vi "Ramp Motors.vi"() -> ()   [LabVIEW 2018]
uses:
  <vilib>/Rock Robotics/WPI/ThirdParty/Phoenix-LabVIEW/Motor Controller/Controls/CTRE_Phoenix_MotorControl_NeutralMode.ctl
  <vilib>/Rock Robotics/WPI/ThirdParty/Phoenix-LabVIEW/Motor Controller/Controls/CTRE_Phoenix_MotorControl_ControlMode.ctl
  Framework/Robot Global Data.vi
  <vilib>/ptbypt/NI_PtbyPt.lvlib
panel:
  in  "Target Time (s)":dbl=0.5
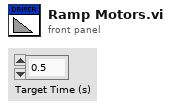
[diagram p1: front panel]
types:
  T1 = typedef "CTRE_Phoenix_MotorControl_NeutralMode.ctl" = enum8{"EEPROMSetting", "Override to Coast", "Override to Brake"}
  T2 = typedef "WPI_MotorControlDeviceRef.ctl" = cluster{"DeviceStatus":errorcluster, "Type":T3, "PWM":cluster{"PWM Channel":T4, "DeadBand":T5}, "CAN":cluster{"Device Number":u8, "SetOutput VI Ref":variant, "GetOutput VI Ref":variant, "Enable VI Ref":variant, "Disable VI Ref":variant, "Data":variant}, "Invert":bool, "DIO PWM":cluster{"PWM \"Enable\" Channel":T4, "DIOChannel":T6, "PWM Rate":dbl}}
  T3 = typedef "WPI_MotorControlType.ctl" = enum16{"PWM", "CAN", "DIO PWM"}
  T4 = typedef "FPGA_DIOPWMChannel.ctl" = enum8{"PWM 0", "PWM 1", "PWM 2", "PWM 3", "PWM 4", "PWM 5", "PWM 6", "PWM 7", "PWM 8", "PWM 9", "PWM MXP 0", "PWM MXP 1", "PWM MXP 2", "PWM MXP 3", "PWM MXP 4", "PWM MXP 5", "PWM MXP 6", "PWM MXP 7", "PWM MXP 8", "PWM MXP 9", "Invalid"}
  T5 = typedef "WPI_PWMDeadband.ctl" = cluster{"Name":string, "maxPositivePwm":i32, "minPositivePwm":i32, "centerPwm":i32, "maxNegativePwm":i32, "minNegativePwm":i32, "angularRange":u16}
  T6 = typedef "FPGA_DIOChannel.ctl" = enum8{"DIO 0", "DIO 1", "DIO 2", "DIO 3", "DIO 4", "DIO 5", "DIO 6", "DIO 7", "DIO 8", "DIO 9", "DIO MXP 0", "DIO MXP 1", "DIO MXP 2", "DIO MXP 3", "DIO MXP 4", "DIO MXP 5", "DIO MXP 6", "DIO MXP 7", "DIO MXP 8", "DIO MXP 9", "DIO MXP 10", "DIO MXP 11", "DIO MXP 12", "DIO MXP 13", "DIO MXP 14", "DIO MXP 15", "SPI Port CS1", "SPI Port CS2", "SPI Port CS3", "SPI Port MISO", "SPI Port MOSI", "Invalid"}
  T7 = typedef "CTRE_Phoenix_MotorControl_ControlMode.ctl" = u16
  T8 = typedef "WPI_DriverStationRobotMode2.ctl" = enum16{"Autonomous Disabled", "Autonomous Enabled", "Teleop Disabled", "Teleop Enabled", "Disconnected", "Finish", "Test Disabled", "Test Enabled", "Emergency Stopped"}
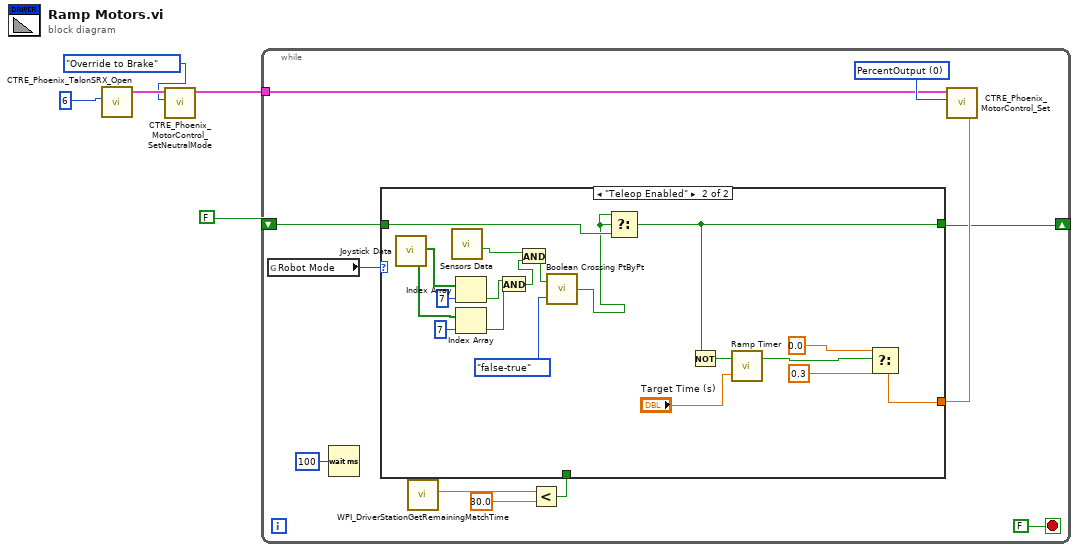
[diagram p0: block diagram]
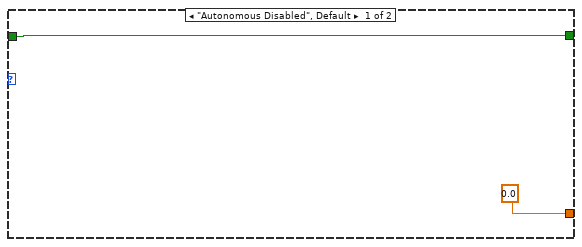
[diagram p2: hidden frame]
diagram:
  n1 = call <vilib>:"CTRE_Phoenix_TalonSRX_Open.vi"("Device Number"=6 ("x")) -> ("CAN Talon SRX Ref"=w4:T2)  [unwired: 9 in, 1 out]
  n2 = call <vilib>:"CTRE_Phoenix_MotorControl_SetNeutralMode.vi"("Motor Control Neutral Mode"=CTRE_Phoenix_MotorControl_NeutralMode."Override to Brake", "PhoenixMotorControlDevRef"=w4) -> ("PhoenixMotorControlDevRef"=w3:T2)  [unwired: 8 in, 1 out]
  n3 = while {
    tunnel: w3 -> [w9]
    shift-right: [w6] -> _
    shift-left: FALSE -> [w7]
    stop <- FALSE stop-if-true
    w14 = T7 0 items=["PercentOutput"=0, "Position"=1, "Velocity"=2, "Current"=3, "Follower"=5, "MotionProfile"=6, "MotionMagic"=7, "MotionProfileArc"=10, "Disabled"=15] ("Control Mode")
    n4 = global read "Robot Global Data.vi" "Robot Mode"() -> (w15:T8)
    n5 = Wait (ms)(milliseconds to wait=u32 100) -> ()  [unwired: 1 out]
    n6 = call <vilib>:"WPI_DriverStationGetRemainingMatchTime.vi"() -> ("Match Time(s)"=w12:sgl)  [unwired: 10 in, 1 out]
    n7 = Less?(x=w12, y=sgl 30.0) -> (x < y?=w10:bool)
    n8 = case shown="\"Teleop Enabled\"" w15 {
      tunnel: w10 -> [_ _]
      tunnel: [sgl 0.0 ("y") w33] -> w8
      tunnel: w7 -> [w17 w32]
      tunnel: [w17 w31] -> w6
      frame "Autonomous Disabled", Default {
      }
      frame "Teleop Enabled" {
        n9 = call "Joystick Data.vi"() -> ("Xbox 360 Out"=w19:bool[], "Xbox One Out"=w20:bool[])  [unwired: 12 in, 6 out]
        n10 = call "Sensors Data.vi"() -> ("Switch Hit Out"=w22:bool)  [unwired: 8 in, 3 out]
        n11 = Index Array(array=w20, index=7) -> (element=w24:bool)
        n12 = Index Array(array=w19, index=7) -> (element=w25:bool)
        n13 = And(x=w24, y=w25) -> (x .and. y?=w23:bool)
        n14 = And(x=w22, y=w23) -> (x .and. y?=w21:bool)
        n15 = call <vilib>:"Boolean Crossing PtByPt.vi"("direction"=enum16{"either", "false-true", "true-false"}."false-true", "input"=w21) -> ("crossing"=w26:bool)  [unwired: 1 in]
        n16 = Select(t=w26, s=w26, f=w32) -> (s? t:f=w31:bool)
        n17 = Not(x=w31) -> (.not. x?=w30:bool)
        n18 = call "Ramp Timer.vi"("Target Time (s)"="Target Time (s)", "Reset Timer"=w30) -> ("Time Reached?"=w27:bool)  [unwired: 1 out]
        n19 = Select(t=0.0, s=w27, f=0.3) -> (s? t:f=w33:dbl)
      }
    }
    n20 = call <vilib>:"CTRE_Phoenix_MotorControl_Set.vi"("Output"=w8, "Control Mode"=w14, "PhoenixMotorControlDevRef"=w9) -> ()  [unwired: 7 in, 2 out]
  }
